vi "NewGame.vi"(8 "error in (no error)":errorcluster, 10 "Engine in":refnum<class "Engine.lvclass">, 11 "DemoGameType (ChildObject)":refnum<class "DemoGame.lvclass">) -> (0 "error out":errorcluster, 2 "Engine out":refnum<class "Engine.lvclass">, 3 "DemoGame out":refnum<class "DemoGame.lvclass">)   [LabVIEW 2019, in "RT_Game.lvlib" / "DemoGame.lvclass"]
uses:
  DemoGame.lvclass
  Engine/Engine.lvclass
  Engine/Coordinate.ctl
  Game/Game.lvclass
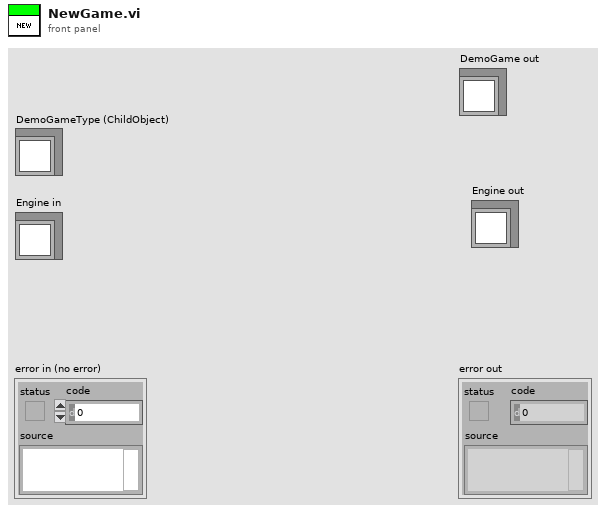
[diagram p1: front panel]
types:
  T1 = typedef "RT_Game.lvlib/Engine.lvclass/Coordinate.ctl" = cluster{"x":dbl, "y":dbl}
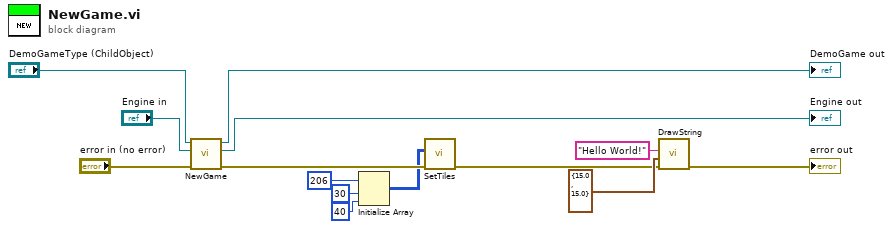
[diagram p0: block diagram]
diagram:
  n1 = call-parent "NewGame.vi"("error in (no error)"="error in (no error)", "Engine in"="Engine in", "GameType (ChildObject)"="DemoGameType (ChildObject)") -> ("error out"=w14:errorcluster, "Engine out"=→"Engine out":refnum<class "Engine.lvclass">, "Game out"=→"DemoGame out":refnum<class "DemoGame.lvclass">)  [unwired: 6 in]
  n2 = Initialize Array(u32 206 ("Numeric"), 30 ("dimension size"), 40 ("dimension size")) -> (w1:u32[][])
  n3 = call "SetTiles.vi"("error in (no error)"=w14, "TileCodes"=w1) -> ("error out"=w5:errorcluster)  [unwired: 9 in]
  n4 = call "DrawString.vi"("error in (no error)"=w5, "Coordinate"=T1 {"x"=15.0, "y"=15.0}, "String"="Hello World!") -> ("error out"=→"error out":errorcluster)  [unwired: 8 in]
